vi "Temperature Converter.vi"() -> ()   [LabVIEW 2018]
panel:
  in  "stop":bool
  in  "Converter":bool
  out "Thermometer (C)":dbl(slide) scale=0.0..100.0
  in  "Temperature (F)":dbl(slide) scale=-50.0..200.0
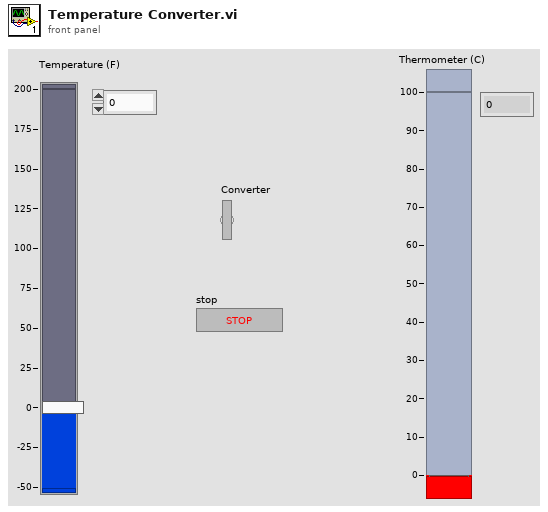
[diagram p1: front panel]
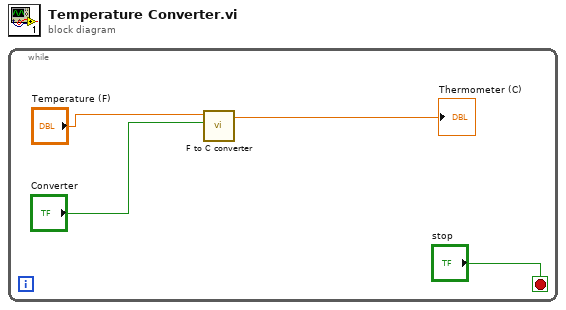
[diagram p0: block diagram]
diagram:
  n1 = while {
    stop <- "stop" stop-if-true
    n2 = call "F to C converter.vi"("Boolean"="Converter", "Temperature (F)"="Temperature (F)") -> ("Numeric"=→"Thermometer (C)":dbl)  [unwired: 9 in]
  }
